vi "PROTECAO.vi"(3 "Estado In":i32) -> (1 "Estado Out":i32)   [LabVIEW 2018]
uses:
  Global_Telescopio.vi
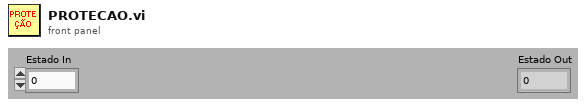
[diagram p1: front panel]
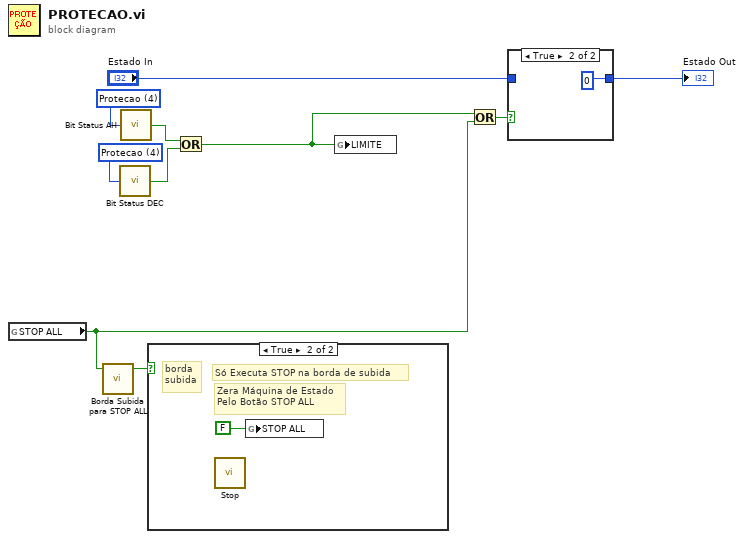
[diagram p0: block diagram]
diagram:
  w9 = u16 4 items=["Alarme", "Atencao", "Erro", "Ocupado", "Protecao", "Embreagem", "Tracking", "Var. Track", "Rápido", "Ligeiro", "Médio", "Lento", "Em movimento", ""] ("NomeStatus")
  w10 = u16 4 items=["Alarme", "Atencao", "Erro", "Ocupado", "Protecao", "Embreagem", "Tracking", "Var. Track", "Rápido", "Ligeiro", "Médio", "Lento", "Em movimento", ""] ("NomeStatus")
  n1 = global read "Global_Telescopio.vi" "STOP ALL"() -> (w3:bool)
  n2 = call "Borda Subida para STOP ALL.vi"("Entrada"=w3) -> ("Boolean"=w2:bool)  [unwired: 4 in]
  n3 = call "Bit Status DEC.vi"("NomeStatus"=w9) -> ("StatBit"=w7:bool)
  n4 = call "Bit Status AH.vi"("NomeStatus"=w10) -> ("StatBit"=w8:bool)
  n5 = case shown="True" w2 {
    frame False {
    }
    frame True {
      # "borda\nsubida"
      # "Zera Máquina de Estado\nPelo Botão STOP ALL"
      # "Só Executa STOP na borda de subida"
      n6 = call "Stop.vi"() -> ()  [unwired: 1 in, 1 out]
      n7 = global write "Global_Telescopio.vi" "STOP ALL"(FALSE ("STOP ALL")) -> ()
    }
  }
  n8 = Or(x=w8, y=w7) -> (x .or. y?=w1:bool)
  n9 = global write "Global_Telescopio.vi" "LIMITE"(w1) -> ()
  n10 = Or(x=w1, y=w3) -> (x .or. y?=w4:bool)
  n11 = case shown="True" w4 {
    tunnel: "Estado In" -> [w12 _]
    tunnel: [w12 0] -> w5
    frame False {
    }
    frame True {
    }
  }
  "Estado Out" <- w5
